vi "SaveHSVComb.vi"(0 "File Name":string, 1 "Intensity":dbl[][](array[numeric]), 2 "intensity_max":dbl, 3 "intensity_min":dbl, 4 "Lifetime":dbl[][](array[numeric]), 5 "lifetime_max (s)":dbl, 6 "lifetime_min (s)":dbl, 7 "error in":errorcluster, 8 "Experiment Name":string, 9 "Index Name":string, 10 "Identify Name":string, 11 "Enable?":bool, 12 "path":path, 14 "Crop Pixels":u16=40, 15 "Time Stamp?":bool) -> (20 "cancelled":bool, 27 "error out":errorcluster)   [LabVIEW 2015]
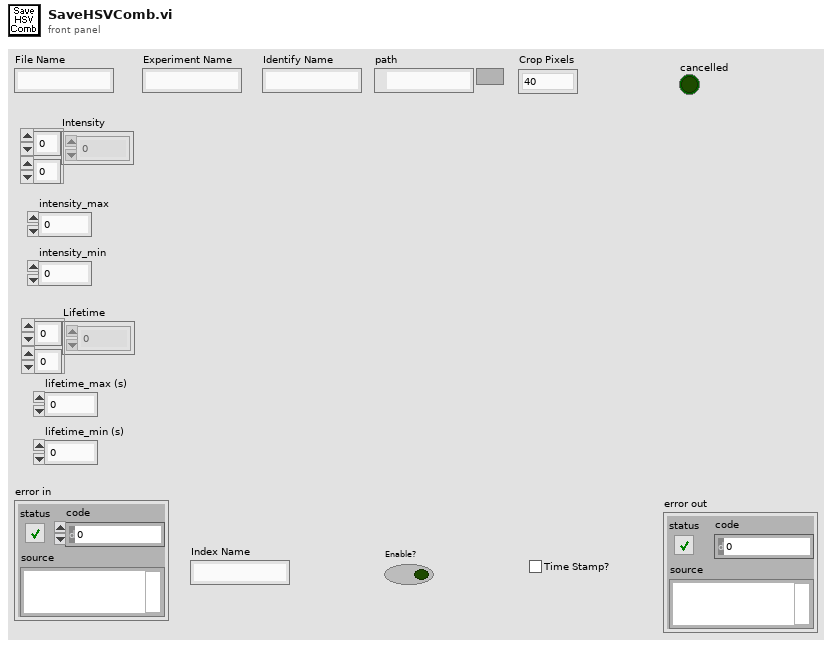
[diagram p1: front panel]
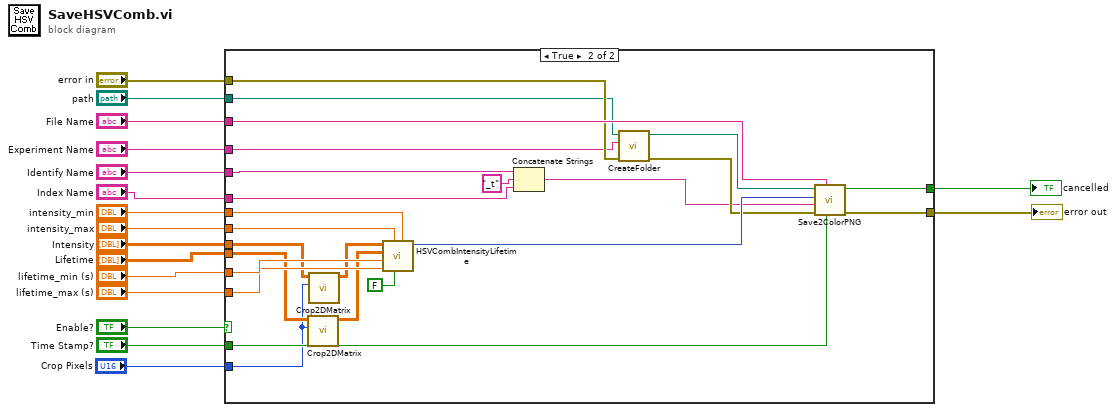
[diagram p0: block diagram]
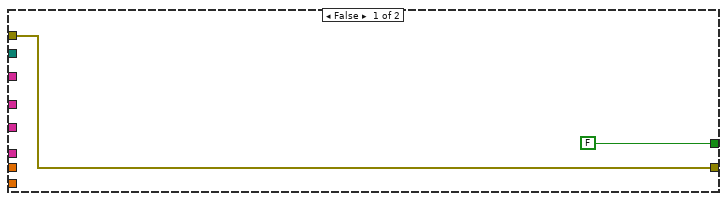
[diagram p2: hidden frame]
diagram:
  n1 = case shown="True" "Enable?" {
    tunnel: "error in" -> [w19 w29]
    tunnel: [w19 w41] -> w16
    tunnel: "Experiment Name" -> [_ w28]
    tunnel: "File Name" -> [_ w42]
    tunnel: "path" -> [_ w27]
    tunnel: [FALSE ("save cancelled") w43] -> w17
    tunnel: "Intensity" -> [_ w34]
    tunnel: "Lifetime" -> [_ w32]
    tunnel: "lifetime_min (s)" -> [_ w40]
    tunnel: "lifetime_max (s)" -> [_ w39]
    tunnel: "intensity_max" -> [_ w38]
    tunnel: "intensity_min" -> [_ w37]
    tunnel: "Identify Name" -> [_ w22]
    tunnel: "Time Stamp?" -> [_ w35]
    tunnel: "Crop Pixels" -> [_ w30]
    tunnel: "Index Name" -> [_ w21]
    frame False {
    }
    frame True {
      n2 = call "Crop2DMatrix.vi"("Crop Pixels"=w30, "Data"=w32) -> ("Cropped Data"=w31:dbl[][])  [unwired: 9 in]
      n3 = call "Crop2DMatrix.vi"("Crop Pixels"=w30, "Data"=w34) -> ("Cropped Data"=w33:dbl[][])  [unwired: 9 in]
      n4 = call "HSVCombIntensityLifetime.vi"("min_intensity"=w37, "Auto Scale?"=FALSE, "max_intensity"=w38, "lifetime_max (s)"=w39, "lifetime_min (s)"=w40, "Lifetime image"=w31, "Intensity image"=w33) -> ("HSV to RGB Picture"=w36:picture)  [unwired: 1 in, 3 out]
      n5 = Concatenate Strings(w22, "_t" ("string"), w21) -> (w20:string)
      n6 = call "CreateFolder.vi"("error in (no error)"=w29, "name"=w28, "base path"=w27) -> ("error out"=w24:errorcluster, "path out"=w25:path)  [unwired: 7 in]
      n7 = call "Save2ColorPNG.vi"("Time Stamp?"=w35, "File Name Prefix"=w42, "error in"=w24, "Identify Name"=w20, "Data Picture"=w36, "Parent Directory"=w25) -> ("error out"=w41:errorcluster, "cancelled"=w43:bool)  [unwired: 4 in]
    }
  }
  "cancelled" <- w17
  "error out" <- w16
